vi "NB_ReadProperty.vi"(8 "error in (no error)":errorcluster, 11 "object in":refnum<class "NativeBaseTemplate.lvclass">) -> (0 "error out":errorcluster, 2 "property":bool, 3 "object out":refnum<class "NativeBaseTemplate.lvclass">)   [LabVIEW 2012, in "NativeBaseTemplate.lvclass"]
uses:
  NativeBaseTemplate.lvclass
  NativeBaseTemplate.lvclass/NativeBaseTemplate.ctl
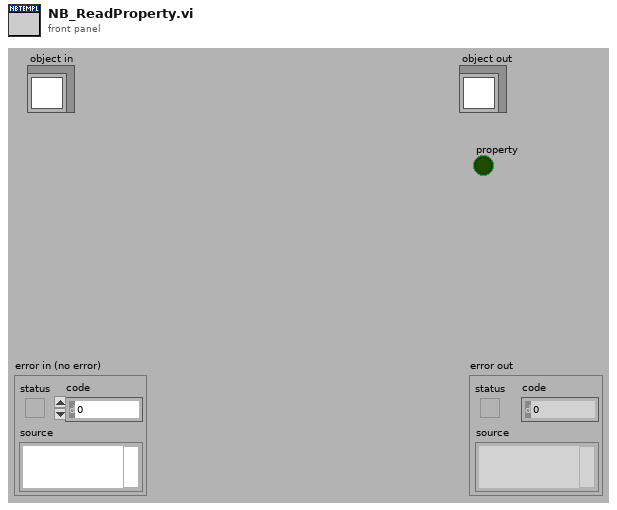
[diagram p1: front panel]
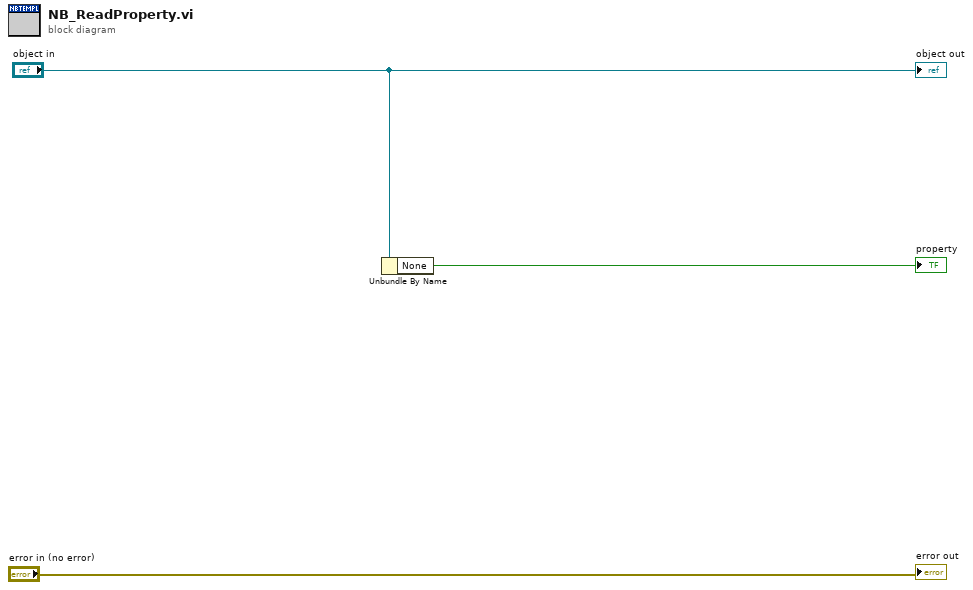
[diagram p0: block diagram]
diagram:
  n1 = Unbundle By Name("object in") -> ("None"=→"property":bool)
  "error out" <- "error in (no error)"
  "object out" <- "object in"
